vi "Close Variable Connections.vi"(11 "Variable References":T1) -> ()   [LabVIEW 2018]
uses:
  Controls/Shared Variable References.ctl
  Controls/VTF Sensors.ctl
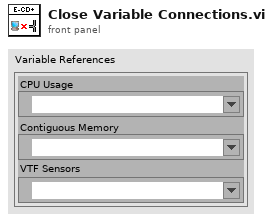
[diagram p1: front panel]
types:
  T1 = typedef "Shared Variable References.ctl" = cluster{"CPU Usage":refnum<k21>, "Contiguous Memory":refnum<k21>, "VTF Sensors":refnum<k21>}
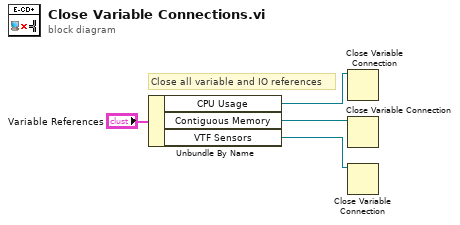
[diagram p0: block diagram]
diagram:
  # "Close all variable and IO references"
  n1 = Unbundle By Name("Variable References") -> ("CPU Usage"=w3:refnum<k21>, "Contiguous Memory"=w4:refnum<k21>, "VTF Sensors"=w1:refnum<k21>)
  n2 = Close Variable Connection(11:w3) -> ()  [unwired: 1 in, 1 out]
  n3 = Close Variable Connection(11:w4) -> ()  [unwired: 1 in, 1 out]
  n4 = Close Variable Connection(11:w1) -> ()  [unwired: 1 in, 1 out]
